vi "SetExternalInterfaces.vi"(8 "ErrorIn":errorcluster, 10 "ExternalInterfaces":T1[](array[typedef]), 11 "ReferenceIn":refnum<class "TemplateGUI.lvclass">) -> (0 "ErrorOut":errorcluster, 3 "ReferenceOut":refnum<class "TemplateGUI.lvclass">)   [LabVIEW 2021, in "TemplateGUIOpenGDSActiveObject.lvlib" / "TemplateGUI.lvclass"]
doc: "Sets the external interface objects that are used by the object. Each interface is defined by:\n\n- the label of the control in the attribute cluster of the object\n\n- the object inself that inherits from the attribute control\n\n- a boolean that indicates if this an array of objects"
uses:
  TemplateGUI.lvclass
  Library_TAF_Support/ClusterArrayConversion/BundledArray.ctl
  0a6ec689-4898-488c-8e07-ed5616c8d135.vi
  0a6ec689-4898-488c-8e07-ed5616c8d135.vi/e733eca7-9823-4359-8665-3b184f9a7377.vi
  0a6ec689-4898-488c-8e07-ed5616c8d135.vi/185eb5ab-e8f7-4395-854b-f566a9b9020c.vi
  <vilib>/Utility/Data Type/Get Cluster Information.vi
  <vilib>/Utility/Data Type/Get Type Information.vi
  <userlib>/_OpenG.lib/lvdata/lvdata.llb/Array of VData to VCluster__ogtk.vi
  <vilib>/Utility/LVClass/Get LV Class Name.vi
  Library_TAF_Support/ClusterArrayConversion/ClusterArrayConversion.lvlib
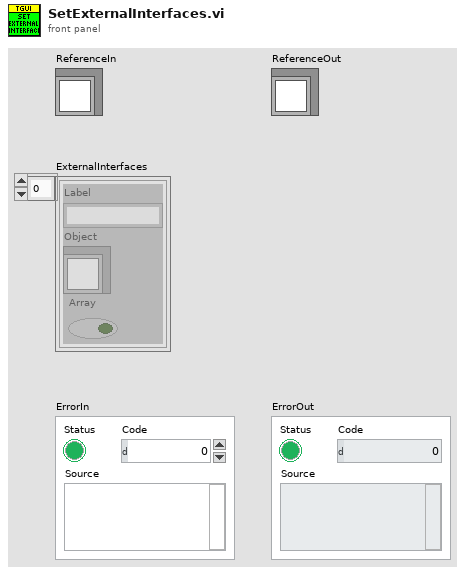
[diagram p1: front panel]
types:
  T1 = typedef "ClusterArrayConversion.lvlib/BundledArray.ctl" = cluster{"Label":string, "Object":refnum<class>, "Array":bool}
  T2 = typedef "TemplateGUI.lvlib/TemplateGUI.lvclass/ObjectAttributes.ctl" = cluster{"Interfaces":cluster{"Dummys":refnum<class>}, "Locals":cluster{"MainGUIActive":refnum<queue>}, "Persistent":cluster{"Dummy":bool}}
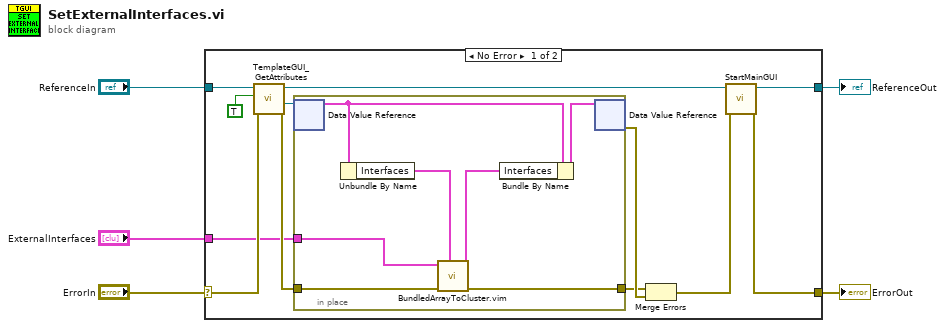
[diagram p0: block diagram]
diagram:
  n1 = case shown="No Error" "ErrorIn" {
    selector: "ErrorIn" -> [w17 w26]
    tunnel: [w12 w26] -> w4
    tunnel: [w6 w25] -> w2
    tunnel: "ReferenceIn" -> [w11 w25]
    tunnel: "ExternalInterfaces" -> [w7 _]
    frame No Error {
      n2 = call "TemplateGUI_GetAttributes.vi"("ErrorIn"=w17, "OnlyGetDvrReference(False)"=TRUE, "ReferenceIn"=w11) -> ("ErrorOut"=w14:errorcluster, "DataRef"=w8:refnum<data-value>, "ReferenceOut"=w10:refnum<class "TemplateGUI.lvclass">)  [unwired: 5 in, 1 out]
      n3 = in-place {
        in-place-border: [w24] -> w15
        in-place-border: w14 -> [w23]
        in-place-border: w7 -> [w18]
        n4 = in-place-dvr #1(w8) -> (w21:T2)  [unwired: 1 out]
        n5 = Unbundle By Name(w21) -> ("Interfaces"=w20:cluster{"Dummys":refnum<class>})
        n6 = call "BundledArrayToCluster.vim"("Type"=w20, "ErrorIn"=w23, "BundeledLabels"=w18) -> ("ErrorOut"=w24:errorcluster, "DataOut"=w19:cluster{"Dummys":refnum<class>})  [unwired: 7 in]
        n7 = Bundle By Name(cluster=w21, "Interfaces"=w19) -> (w22:T2)
        n8 = in-place-dvr #1(w22) -> (w16:errorcluster)  [unwired: 1 out]
      }
      n9 = Merge Errors(w15, w16) -> (w13:errorcluster)
      n10 = call "StartMainGUI.vi"("ErrorIn"=w13, "ReferenceIn"=w10) -> ("ErrorOut"=w12:errorcluster, "ReferenceOut"=w6:refnum<class "TemplateGUI.lvclass">)  [unwired: 6 in, 2 out]
    }
    frame Error {
    }
  }
  "ErrorOut" <- w4
  "ReferenceOut" <- w2
